vi "Constants.vi"() -> (3 "Cluster":T1={"Drive Constants"={"Minumum Feed Forward"=0.085}})   [LabVIEW 2018]
uses:
  ConstantsControl.ctl
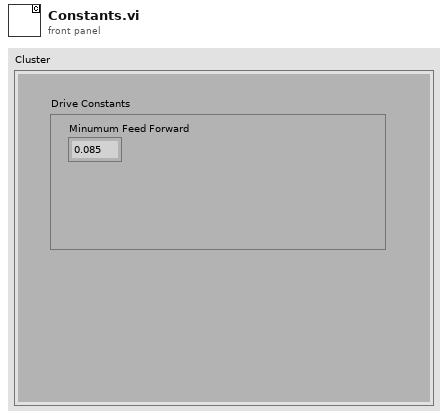
[diagram p1: front panel]
types:
  T1 = typedef "ConstantsControl.ctl" = cluster{"Drive Constants":cluster{"Minumum Feed Forward":dbl}}
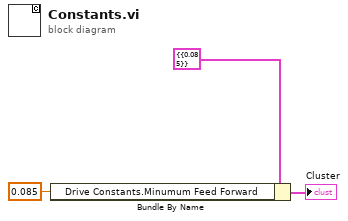
[diagram p0: block diagram]
diagram:
  n1 = Bundle By Name(cluster=T1 {"Drive Constants"={"Minumum Feed Forward"=0.085}} ("Cluster 2"), "Drive Constants.Minumum Feed Forward"=0.085) -> (→"Cluster":T1)
